vi "ElevatorTilt.vi"(10 "Down?":bool=TRUE, 11 "Up":bool=TRUE) -> ()   [LabVIEW 2017]
uses:
  <vilib>/Rock Robotics/WPI/Solenoid/WPI_SolenoidValue.ctl
  <vilib>/Rock Robotics/WPI/Solenoid/WPI_SolenoidSetEnum.vi
panel:
  in  "Boolean":bool
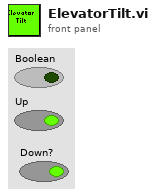
[diagram p1: front panel]
types:
  T1 = typedef "WPI_SolenoidValue.ctl" = enum16{"Off", "On", "Forward", "Reverse"}
  T2 = typedef "WPI_SolenoidDevRef.ctl" = cluster{"DevStatus":errorcluster, "Pneumatics Control Module":u8, "Forward Solenoid Channel":T3, "Reverse Solenoid Channel":T3}
  T3 = typedef "WPI_SolenoidChannel.ctl" = enum8{"Solenoid 0", "Solenoid 1", "Solenoid 2", "Solenoid 3", "Solenoid 4", "Solenoid 5", "Solenoid 6", "Solenoid 7", "Invalid"}
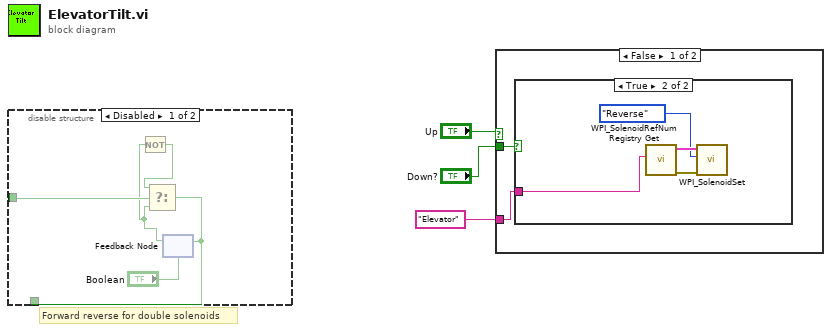
[diagram p0: block diagram]
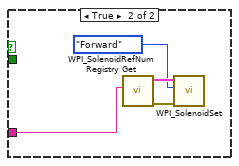
[diagram p3: hidden frame]
diagram:
  # "Forward reverse for double solenoids"
  n1 = disable-structure shown="Disabled" {
    disable-tunnel: _ -> [w8 _]
    disable-tunnel: [w4 _] -> _
    frame Disabled {
      n2 = feedback #1("Boolean") -> (w7:bool)
      n3 = Not(x=w7) -> (.not. x?=w6:bool)
      n4 = Select(t=w6, s=w8, f=w7) -> (s? t:f=w4:bool)
      n5 = feedback-in #1(w4) -> ()
    }
    frame Enabled {
    }
  }
  n6 = case shown="False" "Up" {
    tunnel: "Down?" -> [w10 _]
    tunnel: "Elevator" ("refnum name") -> [w9 w15]
    frame False {
      n7 = case shown="True" w10 {
        tunnel: w9 -> [_ w11]
        frame False {
        }
        frame True {
          n8 = call <vilib>:"WPI_SolenoidRefNum Registry Get.vi"("refnum name"=w11) -> ("error out"=w13:errorcluster, "SolenoidDevRef"=w14:T2)  [unwired: 9 in]
          n9 = call-poly <vilib>:"WPI_SolenoidSet.vi"("error in (no error)"=w13, "Value"=WPI_SolenoidValue."Reverse", "SolenoidDevRef"=w14) -> ()  [unwired: 7 in, 2 out]
        }
      }
    }
    frame True {
      n10 = call <vilib>:"WPI_SolenoidRefNum Registry Get.vi"("refnum name"=w15) -> ("error out"=w17:errorcluster, "SolenoidDevRef"=w18:T2)  [unwired: 9 in]
      n11 = call-poly <vilib>:"WPI_SolenoidSet.vi"("error in (no error)"=w17, "Value"=WPI_SolenoidValue."Forward", "SolenoidDevRef"=w18) -> ()  [unwired: 7 in, 2 out]
    }
  }
